vi "Finish.vi"   [LabVIEW 2015]
doc: "This VI is called just before exiting. It is expected to close I/O refnum, save collected data, etc."
uses:
  <vilib>/Rock Robotics/WPI/Utilities/WPI_GetSetVariantRefNum.vi
types:
  T1 = typedef "WPI_JoystickDevRef.ctl" = cluster{"Device":T2}
  T2 = typedef "WPI_JoystickDeviceEnum.ctl" = enum16{"USB 0", "USB 1", "USB 2", "USB 3", "USB 4", "USB 5"}
  T3 = typedef "WPI_SolenoidDevRef.ctl" = cluster{"DevStatus":errorcluster, "Pneumatics Control Module":u8, "Forward Solenoid Channel":T4, "Reverse Solenoid Channel":T4}
  T4 = typedef "WPI_SolenoidChannel.ctl" = enum8{"Solenoid 0", "Solenoid 1", "Solenoid 2", "Solenoid 3", "Solenoid 4", "Solenoid 5", "Solenoid 6", "Solenoid 7", "Invalid"}
  T5 = typedef "WPI_CompressorDevRef.ctl" = cluster{"DevStatus":errorcluster, "Pneumatics Control Module":u8}
  T6 = typedef "WPI_EncoderDevRef.ctl" = cluster{"DevStatus":errorcluster, "EncoderIndex":T7, "CounterIndex":T8, "DistancePerCount":dbl, "Decoding Type":T9}
  T7 = typedef "FPGA_EncoderIdx.ctl" = enum8{"Enc 0", "Enc 1", "Enc 2", "Enc 3", "Enc 4", "Enc 5", "Enc 6", "Enc 7", "Invalid"}
  T8 = typedef "FPGA_CounterCtrSystemIndex.ctl" = enum8{"Ctr 0", "Ctr 1", "Ctr 2", "Ctr 3", "Ctr 4", "Ctr 5", "Ctr 6", "Ctr 7", "Invalid"}
  T9 = typedef "WPI_EncoderType.ctl" = enum16{"1x", "2x", "4x"}
  T10 = typedef "WPI_MotorControlDeviceRef.ctl" = cluster{"DeviceStatus":errorcluster, "Type":T11, "PWM":cluster{"PWM Channel":T12, "DeadBand":T13}, "CAN":cluster{"Device Number":u8, "Control Mode":T14, "Semaphore":T15, "Max Vout":dbl, "TalonSRX Control Mode":T16}, "Invert":bool}
  T11 = typedef "WPI_MotorControlType.ctl" = enum16{"PWM", "CAN", "CANTalonSRX"}
  T12 = typedef "FPGA_DIOPWMChannel.ctl" = enum8{"PWM 0", "PWM 1", "PWM 2", "PWM 3", "PWM 4", "PWM 5", "PWM 6", "PWM 7", "PWM 8", "PWM 9", "PWM MXP 0", "PWM MXP 1", "PWM MXP 2", "PWM MXP 3", "PWM MXP 4", "PWM MXP 5", "PWM MXP 6", "PWM MXP 7", "PWM MXP 8", "PWM MXP 9", "Invalid"}
  T13 = typedef "WPI_PWMDeadband.ctl" = cluster{"Name":string, "maxPositivePwm":i32, "minPositivePwm":i32, "centerPwm":i32, "maxNegativePwm":i32, "minNegativePwm":i32, "angularRange":u16}
  T14 = typedef "WPI_CANJaguar_ControlMode.ctl" = enum8{"Percent VBus", "Current", "Speed", "Position", "Voltage"}
  T15 = typedef "Semaphore RefNum" = refnum<k1>
  T16 = typedef "WPI_CANTalonSRX_APIControlMode.ctl" = enum8{"Percent VBus", "Speed", "Position", "Slave", "Unchanged / Invalid", "Voltage Compensation", "Current", "Motion Profile"}
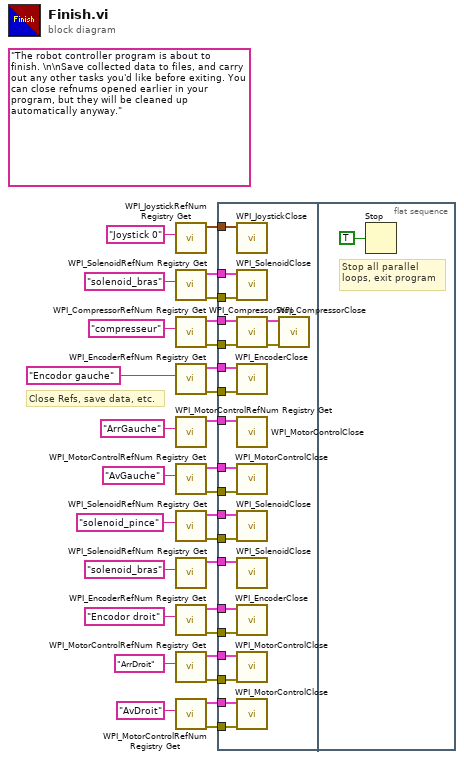
[diagram p0: block diagram]
diagram:
  (unwired) "The robot controller program is about to finish. \n\nSave collected data to files, and carry out any other tasks you'd like before exiting. You can close refnums opened earlier in your program, but they will be cleaned up automatically anyway."
  # "Close Refs, save data, etc."
  n1 = call <vilib>:"WPI_JoystickRefNum Registry Get.vi"("refnum name"="Joystick 0") -> ("JoystickDevRef"=w29:T1)  [unwired: 1 in, 9 out]
  n2 = call <vilib>:"WPI_SolenoidRefNum Registry Get.vi"("refnum name"="solenoid_bras") -> ("error out"=w14:errorcluster, "SolenoidDevRef"=w28:T3)  [unwired: 9 in]
  n3 = call <vilib>:"WPI_CompressorRefNum Registry Get.vi"("refnum name"="compresseur") -> ("error out"=w23:errorcluster, "CompressorDevRef"=w24:T5)  [unwired: 9 in]
  n4 = call <vilib>:"WPI_EncoderRefNum Registry Get.vi"("refnum name"="Encodor gauche") -> ("error out"=w18:errorcluster, "EncoderDevRef"=w19:T6)  [unwired: 9 in]
  n5 = call <vilib>:"WPI_MotorControlRefNum Registry Get.vi"("refnum name"="ArrGauche") -> ("MotorControlDevRef"=w11:T10)  [unwired: 9 in, 1 out]
  n6 = call <vilib>:"WPI_MotorControlRefNum Registry Get.vi"("refnum name"="AvGauche") -> ("error out"=w7:errorcluster, "MotorControlDevRef"=w13:T10)  [unwired: 9 in]
  n7 = call <vilib>:"WPI_SolenoidRefNum Registry Get.vi"("refnum name"="solenoid_pince") -> ("error out"=w15:errorcluster, "SolenoidDevRef"=w25:T3)  [unwired: 9 in]
  n8 = call <vilib>:"WPI_SolenoidRefNum Registry Get.vi"("refnum name"="solenoid_bras") -> ("SolenoidDevRef"=w1:T3)  [unwired: 9 in, 1 out]
  n9 = call <vilib>:"WPI_EncoderRefNum Registry Get.vi"("refnum name"="Encodor droit") -> ("error out"=w17:errorcluster, "EncoderDevRef"=w16:T6)  [unwired: 9 in]
  n10 = call <vilib>:"WPI_MotorControlRefNum Registry Get.vi"("refnum name"="ArrDroit") -> ("error out"=w8:errorcluster, "MotorControlDevRef"=w12:T10)  [unwired: 9 in]
  n11 = call <vilib>:"WPI_MotorControlRefNum Registry Get.vi"("refnum name"="AvDroit") -> ("error out"=w9:errorcluster, "MotorControlDevRef"=w10:T10)  [unwired: 9 in]
  n12 = flat-sequence {
    tunnel: w29 -> [w51]
    tunnel: w28 -> [w50]
    tunnel: w25 -> [w49]
    tunnel: w24 -> [w46]
    tunnel: w23 -> [w45]
    tunnel: w19 -> [w44]
    tunnel: w18 -> [w43]
    tunnel: w17 -> [w42]
    tunnel: w16 -> [w41]
    tunnel: w15 -> [w40]
    tunnel: w14 -> [w39]
    tunnel: w13 -> [w38]
    tunnel: w12 -> [w37]
    tunnel: w11 -> [w36]
    tunnel: w10 -> [w35]
    tunnel: w9 -> [w34]
    tunnel: w8 -> [w33]
    tunnel: w7 -> [w32]
    tunnel: w1 -> [w31]
    frame #0 {
      n13 = call <vilib>:"WPI_JoystickClose.vi"("JoystickDevRef"=w51) -> ()  [unwired: 11 out]
      n14 = call <vilib>:"WPI_SolenoidClose.vi"("error in (no error)"=w39, "SolenoidDevRef"=w50) -> ()  [unwired: 9 in, 1 out]
      n15 = call <vilib>:"WPI_CompressorStop.vi"("error in (no error)"=w45, "CompressorDevRef"=w46) -> ("error out"=w48:errorcluster, "CompressorDevRef"=w47:T5)  [unwired: 8 in]
      n16 = call <vilib>:"WPI_EncoderClose.vi"("error in (no error)"=w43, "EncoderDevRef"=w44) -> ()  [unwired: 9 in, 1 out]
      n17 = call <vilib>:"WPI_MotorControlClose.vi"("MotorControlDevRef"=w36) -> ()  [unwired: 10 in, 1 out]
      n18 = call <vilib>:"WPI_MotorControlClose.vi"("error in (no error)"=w32, "MotorControlDevRef"=w38) -> ()  [unwired: 9 in, 1 out]
      n19 = call <vilib>:"WPI_SolenoidClose.vi"("error in (no error)"=w40, "SolenoidDevRef"=w49) -> ()  [unwired: 9 in, 1 out]
      n20 = call <vilib>:"WPI_SolenoidClose.vi"("SolenoidDevRef"=w31) -> ()  [unwired: 10 in, 1 out]
      n21 = call <vilib>:"WPI_EncoderClose.vi"("error in (no error)"=w42, "EncoderDevRef"=w41) -> ()  [unwired: 9 in, 1 out]
      n22 = call <vilib>:"WPI_MotorControlClose.vi"("error in (no error)"=w33, "MotorControlDevRef"=w37) -> ()  [unwired: 9 in, 1 out]
      n23 = call <vilib>:"WPI_MotorControlClose.vi"("error in (no error)"=w34, "MotorControlDevRef"=w35) -> ()  [unwired: 9 in, 1 out]
      n24 = call <vilib>:"WPI_CompressorClose.vi"("error in (no error)"=w48, "CompressorDevRef"=w47) -> ()  [unwired: 9 in, 1 out]
    }
    frame #1 {
      # "Stop all parallel\nloops, exit program"
      n25 = Stop(stop? (T)=TRUE ("Quit")) -> ()
    }
  }
